vi "TwoSensorMagazineLogic.vi"(4 "Outtake Side Sensor":bool, 5 "Intake Side Sensor":bool, 6 "Outtake Button":bool, 7 "Intake Toggle":bool) -> (0 "Intake Pistons":bool, 1 "Kicker Motors":dbl, 2 "Magazine Motors":dbl, 3 "Intake Motors":dbl)   [LabVIEW 2020]
uses:
  MagazineControl.ctl
  TitanLib/Lib/TitanLib.lvlib
panel:
  out "Current State":T1
  in  "Kicker Power":dbl=0.5
  in  "Magazine Power":dbl=1.0
  in  "Input Power":dbl=1.0
  in  "Initial State":T1
  # "Inputs"
  # "Power Levels"
  # "Outputs"
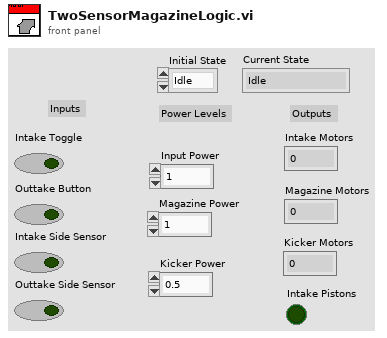
[diagram p1: front panel]
types:
  T1 = typedef "MagazineControl.ctl" = enum16{"Idle", "Intaking", "Outtake", "One Ball", "One Ball Intake", "One Ball Outtake", "Two Balls", "Two Ball Outtake"}
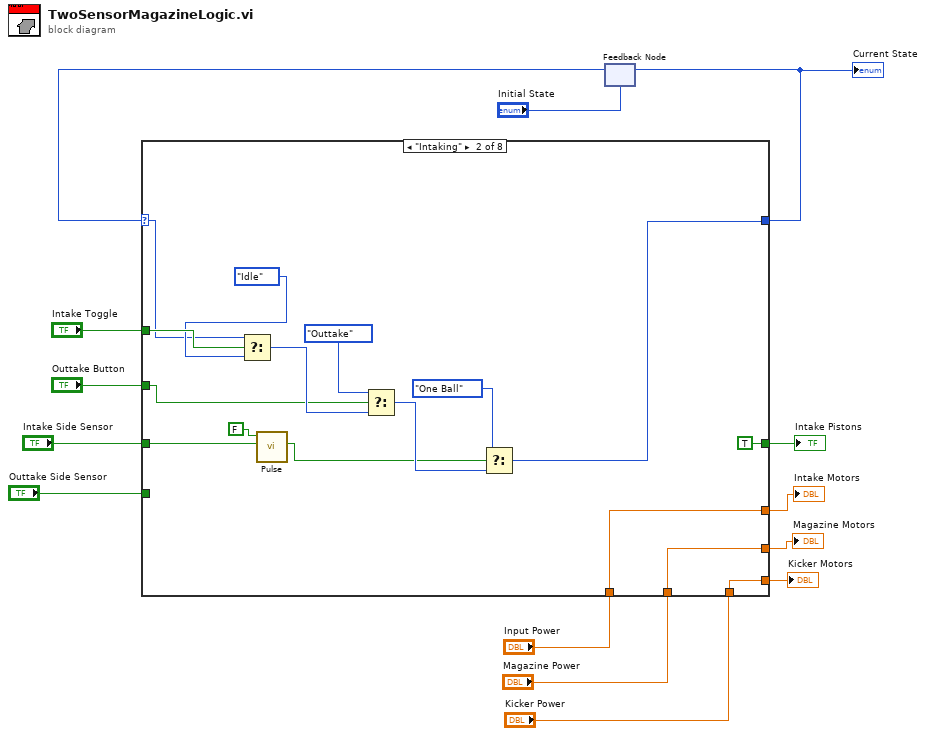
[diagram p0: block diagram]
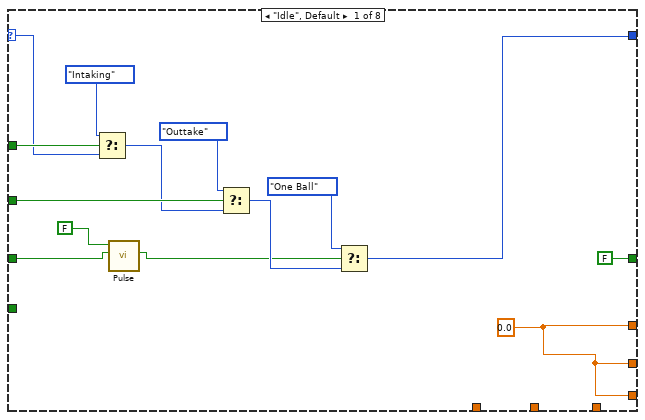
[diagram p2: hidden frame]
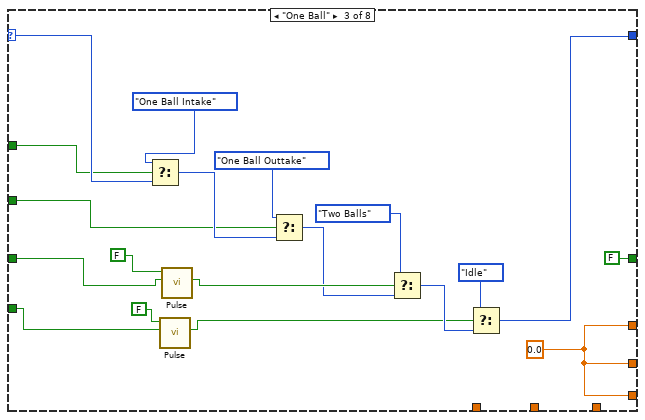
[diagram p3: hidden frame]
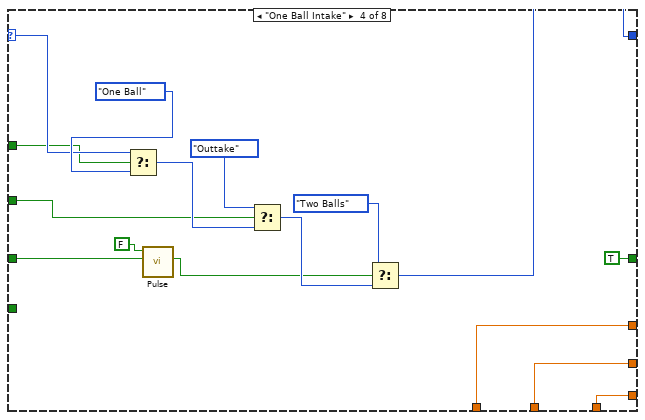
[diagram p4: hidden frame]
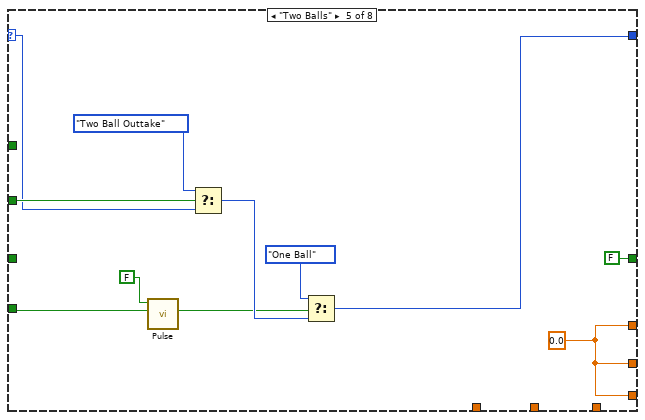
[diagram p5: hidden frame]
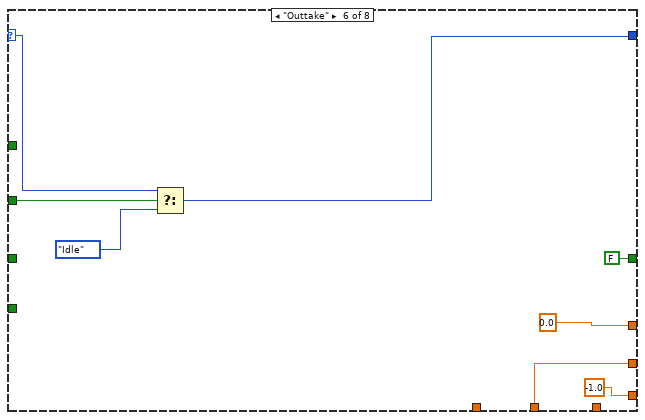
[diagram p6: hidden frame]
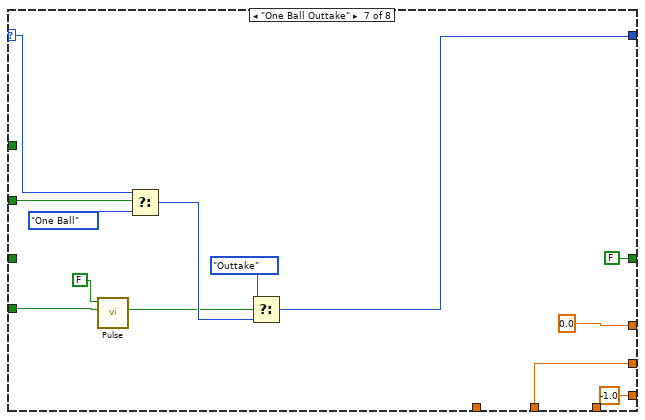
[diagram p7: hidden frame]
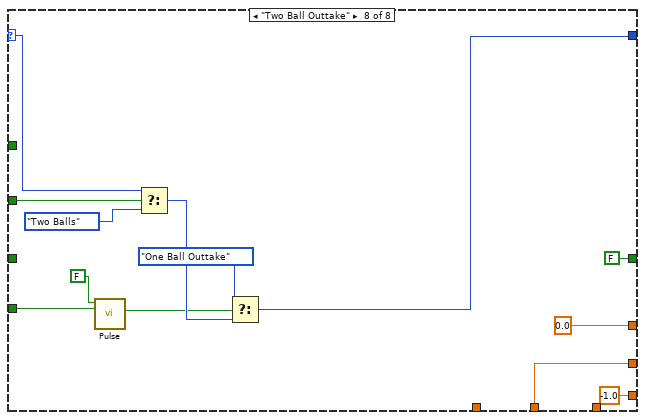
[diagram p8: hidden frame]
diagram:
  n1 = feedback #1("Initial State") -> (w3:T1)
  n2 = case shown="\"Intaking\"" w3 {
    selector: w3 -> [w24 w36 w54 w69 w89 w97 w107 w120]
    tunnel: "Intake Toggle" -> [w28 w39 w53 w68 _ _ _ _]
    tunnel: "Outtake Button" -> [w27 w38 w55 w70 w90 w98 w108 w121]
    tunnel: "Intake Side Sensor" -> [w18 w32 w56 w71 _ _ _ _]
    tunnel: [w20 w40 w49 w72 w86 w95 w103 w116] -> w2
    tunnel: [w16 w35 w52 w67 w87 0.0 ("Input Power") 0.0 ("Input Power") 0.0 ("Input Power")] -> w9
    tunnel: "Input Power" -> [_ w35 _ w67 _ _ _ _]
    tunnel: [w16 w34 w52 w66 w87 w92 w111 w124] -> w11
    tunnel: "Magazine Power" -> [_ w34 _ w66 _ w92 w111 w124]
    tunnel: [w16 w30 w52 w65 w87 -1.0 ("Kicker Motors") -1.0 ("Kicker Motors") -1.0 ("Kicker Motors")] -> w13
    tunnel: "Kicker Power" -> [_ w30 _ w65 _ _ _ _]
    tunnel: "Outtake Side Sensor" -> [_ _ w47 _ w82 _ w101 w115]
    tunnel: [FALSE ("Intake Pistons") TRUE ("Intake Pistons") FALSE ("Intake Pistons") TRUE ("Intake Pistons") FALSE ("Intake Pistons") FALSE ("Intake Pistons") FALSE ("Intake Pistons") FALSE ("Intake Pistons")] -> w1
    frame "Idle", Default {
      w16 = 0.0 ("Input Power")
      n3 = Select(t=MagazineControl."Intaking", s=w28, f=w24) -> (s? t:f=w26:T1)
      n4 = call "Pulse.vi"("Input"=w18, "Rising Edge?"=FALSE) -> ("Output"=w19:bool)  [unwired: 9 in]
      n5 = Select(t=MagazineControl."Outtake", s=w27, f=w26) -> (s? t:f=w25:T1)
      n6 = Select(t=MagazineControl."One Ball", s=w19, f=w25) -> (s? t:f=w20:T1)
    }
    frame "Intaking" {
      n7 = Select(t=w36, s=w39, f=MagazineControl."Idle" ("t")) -> (s? t:f=w43:T1)
      n8 = call "Pulse.vi"("Input"=w32, "Rising Edge?"=FALSE) -> ("Output"=w33:bool)  [unwired: 9 in]
      n9 = Select(t=MagazineControl."Outtake", s=w38, f=w43) -> (s? t:f=w44:T1)
      n10 = Select(t=MagazineControl."One Ball", s=w33, f=w44) -> (s? t:f=w40:T1)
    }
    frame "One Ball" {
      w52 = 0.0 ("Input Power")
      n11 = Select(t=MagazineControl."One Ball Intake", s=w53, f=w54) -> (s? t:f=w61:T1)
      n12 = call "Pulse.vi"("Input"=w47, "Rising Edge?"=FALSE) -> ("Output"=w46:bool)  [unwired: 9 in]
      n13 = call "Pulse.vi"("Input"=w56, "Rising Edge?"=FALSE) -> ("Output"=w63:bool)  [unwired: 9 in]
      n14 = Select(t=MagazineControl."One Ball Outtake", s=w55, f=w61) -> (s? t:f=w62:T1)
      n15 = Select(t=MagazineControl."Two Balls", s=w63, f=w62) -> (s? t:f=w51:T1)
      n16 = Select(t=MagazineControl."Idle", s=w46, f=w51) -> (s? t:f=w49:T1)
    }
    frame "One Ball Intake" {
      n17 = Select(t=w69, s=w68, f=MagazineControl."One Ball" ("t")) -> (s? t:f=w78:T1)
      n18 = call "Pulse.vi"("Input"=w71, "Rising Edge?"=FALSE) -> ("Output"=w74:bool)  [unwired: 9 in]
      n19 = Select(t=MagazineControl."Outtake", s=w70, f=w78) -> (s? t:f=w79:T1)
      n20 = Select(t=MagazineControl."Two Balls", s=w74, f=w79) -> (s? t:f=w72:T1)
    }
    frame "Two Balls" {
      w87 = 0.0 ("Input Power")
      n21 = call "Pulse.vi"("Input"=w82, "Rising Edge?"=FALSE) -> ("Output"=w83:bool)  [unwired: 9 in]
      n22 = Select(t=MagazineControl."Two Ball Outtake", s=w90, f=w89) -> (s? t:f=w85:T1)
      n23 = Select(t=MagazineControl."One Ball", s=w83, f=w85) -> (s? t:f=w86:T1)
    }
    frame "Outtake" {
      n24 = Select(t=w97, s=w98, f=MagazineControl."Idle") -> (s? t:f=w95:T1)
    }
    frame "One Ball Outtake" {
      n25 = call "Pulse.vi"("Input"=w101, "Rising Edge?"=FALSE) -> ("Output"=w102:bool)  [unwired: 9 in]
      n26 = Select(t=w107, s=w108, f=MagazineControl."One Ball") -> (s? t:f=w105:T1)
      n27 = Select(t=MagazineControl."Outtake", s=w102, f=w105) -> (s? t:f=w103:T1)
    }
    frame "Two Ball Outtake" {
      n28 = call "Pulse.vi"("Input"=w115, "Rising Edge?"=FALSE) -> ("Output"=w114:bool)  [unwired: 9 in]
      n29 = Select(t=w120, s=w121, f=MagazineControl."Two Balls") -> (s? t:f=w118:T1)
      n30 = Select(t=MagazineControl."One Ball Outtake", s=w114, f=w118) -> (s? t:f=w116:T1)
    }
  }
  "Intake Motors" <- w9
  "Magazine Motors" <- w11
  "Kicker Motors" <- w13
  "Current State" <- w2
  "Intake Pistons" <- w1
  n31 = feedback-in #1(w2) -> ()
